vi "stop.vi"(8 "error in (no error)":errorcluster, 11 "Glaz-I in":refnum<class "Glaz.lvclass">) -> (0 "error out":errorcluster, 3 "Glaz-I out":refnum<class "Glaz.lvclass">)   [LabVIEW 2019, in "Glaz.lvclass"]
uses:
  Glaz.lvclass
  _cameraBase/_cameraBase.lvclass
  <userlib>/GlazLabView/GlazLib.lvlib
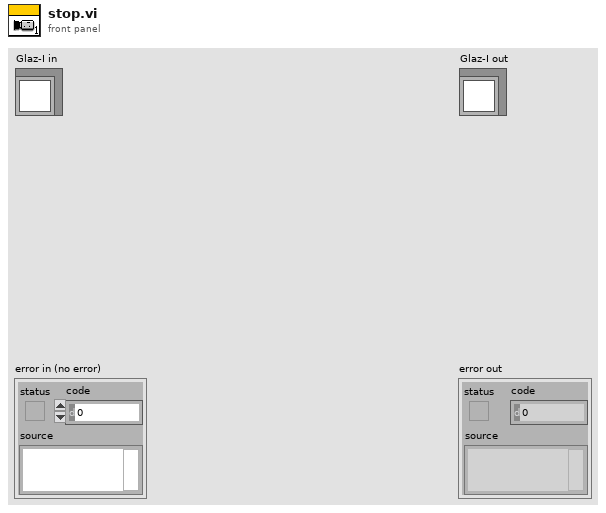
[diagram p1: front panel]
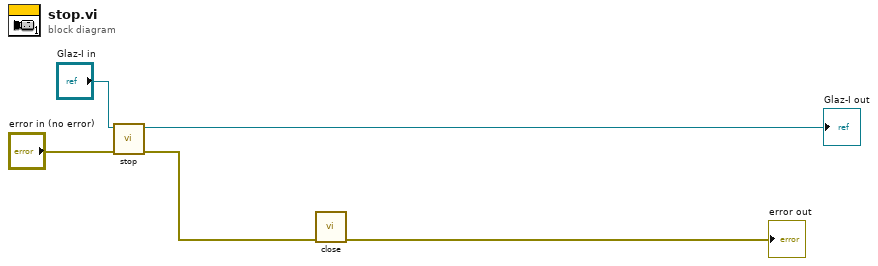
[diagram p0: block diagram]
diagram:
  n1 = call-parent "stop.vi"("error in (no error)"="error in (no error)", "_cameraBase in"="Glaz-I in") -> ("error out"=w2:errorcluster, "_cameraBase out"=→"Glaz-I out":refnum<class "Glaz.lvclass">)  [unwired: 8 in]
  n2 = call <userlib>:"close.vi"("error in (no error)"=w2) -> ("error out"=→"error out":errorcluster)  [unwired: 9 in, 1 out]
